vi "_add_to_header_maps.vi"(10 "ordered headers":cluster{"header":string, "value":string}[](array[cluster]), 11 "httpHeaders in":refnum<class "httpHeaders.lvclass">) -> (3 "httpHeaders out":refnum<class "httpHeaders.lvclass">)   [LabVIEW 2020, in "httpClient.lvlib" / "httpHeaders.lvclass"]
uses:
  httpHeaders.lvclass
  httpHeaders.lvclass/httpHeaders.ctl
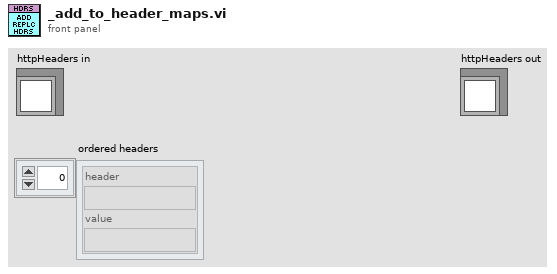
[diagram p1: front panel]
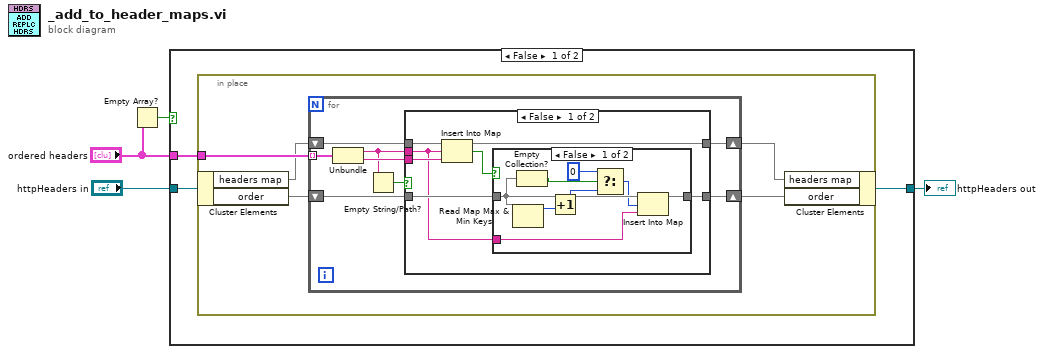
[diagram p0: block diagram]
diagram:
  n1 = Empty Array?(array="ordered headers") -> (empty?=w1:bool)
  n2 = case shown="False" w1 {
    tunnel: "httpHeaders in" -> [w7 w39]
    tunnel: [w6 w39] -> w3
    tunnel: "ordered headers" -> [w5 _]
    frame False {
      n3 = in-place {
        in-place-border: w5 -> [w12]
        n4 = in-place-cluster #1(w7) -> ("headers map"=w11:map{string, string}, "order"=w10:map{i32, string})
        n5 = for {
          tunnel: w12 -> [w20] mode=indexing
          shift-right: [w15] -> w9
          shift-left: w11 -> [w19]
          shift-right: [w16] -> w8
          shift-left: w10 -> [w17]
          n6 = Unbundle(w20) -> ("header"=w14:string, "value"=w18:string)
          n7 = Empty String/Path?(string/path=w14) -> (empty?=w13:bool)
          n8 = case shown="False" w13 {
            tunnel: w19 -> [w27 w38]
            tunnel: w18 -> [w26 _]
            tunnel: w17 -> [w24 w37]
            tunnel: [w23 w37] -> w16
            tunnel: [w22 w38] -> w15
            tunnel: w14 -> [w21 _]
            frame False {
              n9 = Insert Into Map(map in=w27, key=w21, value=w26) -> (map out=w22:map{string, string}, key already included?=w25:bool)  [unwired: 1 out]
              n10 = case shown="False" w25 {
                tunnel: w21 -> [w33 _]
                tunnel: w24 -> [w32 w36]
                tunnel: [w34 w36] -> w23
                frame False {
                  n11 = Read Map Max & Min Keys(11:w32) -> (3:w35:i32)  [unwired: 1 out]
                  n12 = Empty Collection?(1:w32) -> (0:w31:bool)
                  n13 = Increment(x=w35) -> (x+1=w30:i32)
                  n14 = Select(t=0, s=w31, f=w30) -> (s? t:f=w29:i32)
                  n15 = Insert Into Map(map in=w32, key=w29, value=w33) -> (map out=w34:map{i32, string})  [unwired: 2 out]
                }
                frame True {
                  # "Already included.\nNo action on ordering"
                }
              }
            }
            frame True {
              # "Skip empty header name"
            }
          }
        }
        n16 = in-place-cluster #1("headers map"=w9, "order"=w8) -> (w6:refnum<class "httpHeaders.lvclass">)
      }
    }
    frame True {
      # "empty input"
    }
  }
  "httpHeaders out" <- w3
